vi "Warn.vi"(8 "NwarnIN":bool, 9 "HwarnIN":bool, 10 "warncontN":T1={"alarmliqN"=90.0, "warn?N"=FALSE, "lessthan?N"=FALSE}, 11 "warncontHe":T2={"alarmliqHe"=85.0, "warn?He"=FALSE, "lessthan?He"=FALSE}) -> (2 "warnNOUT":T1={"alarmliqN"=90.0, "warn?N"=FALSE, "lessthan?N"=FALSE}, 3 "warnHeOUT":T2={"alarmliqHe"=85.0, "warn?He"=FALSE, "lessthan?He"=FALSE})   [LabVIEW 2009, in "Level Meter.lvclass"]
uses:
  Level Meter.lvclass
  Global/Sound Files.vi
panel:
  in  "turnoff":bool
  out "Nwarn":bool caption="LN"
  out "Hwarn":bool caption="LHe"
  in  "exit":bool
  out "disp":string
  out "warn2":bool
  out "warn1":bool
  # "Off"
  # "On"
  # "Greater"
  # "Less"
  # "Off"
  # "On"
  # "Greater"
  # "Less"
  # "Off"
  # "On"
  # "Greater"
  # "Less"
  # "Off"
  # "On"
  # "Greater"
  # "Less"
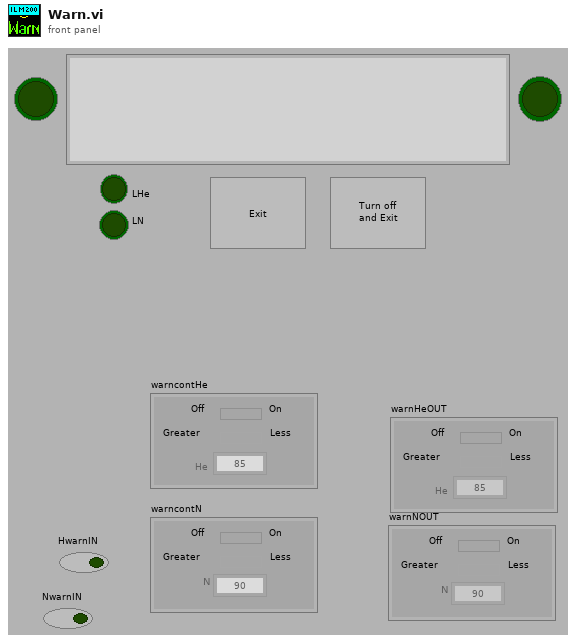
[diagram p1: front panel]
types:
  T1 = cluster{"alarmliqN":dbl, "warn?N":bool, "lessthan?N":bool}
  T2 = cluster{"alarmliqHe":dbl, "warn?He":bool, "lessthan?He":bool}
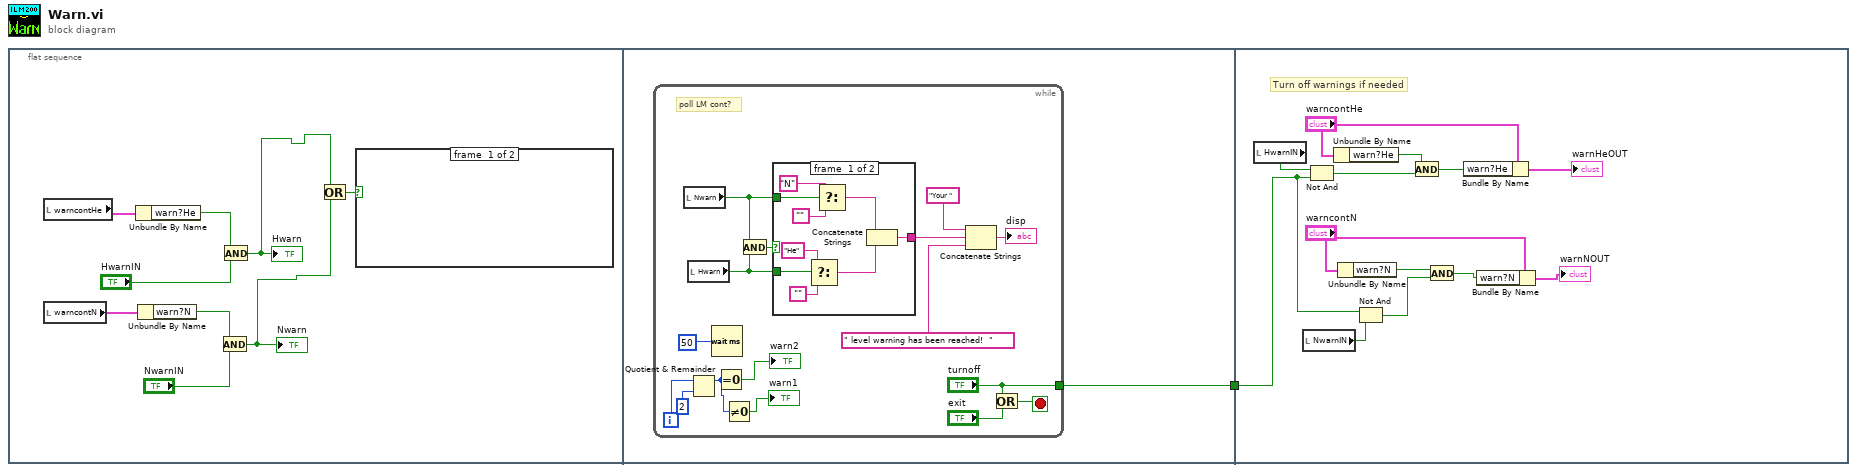
[diagram p0: block diagram]
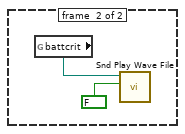
[diagram p2: hidden frame]
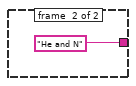
[diagram p3: hidden frame]
diagram:
  n1 = flat-sequence {
    tunnel: [w13] -> w1
    tunnel: w1 -> [w42]
    frame #0 {
      n2 = local read "warncontHe"() -> (w10:T2)
      n3 = local read "warncontN"() -> (w6:T1)
      n4 = Unbundle By Name(w10) -> ("warn?He"=w9:bool)
      n5 = Unbundle By Name(w6) -> ("warn?N"=w7:bool)
      n6 = And(x=w7, y="NwarnIN") -> (x .and. y?=w2:bool)
      "Nwarn" <- w2
      n7 = And(x=w9, y="HwarnIN") -> (x .and. y?=w3:bool)
      "Hwarn" <- w3
      n8 = Or(x=w3, y=w2) -> (x .or. y?=w4:bool)
      n9 = case shown="True" w4 {
        frame #0 {
        }
        frame #1 {
          n10 = global read "Sound Files.vi" "battcrit"() -> (w11:path)
          n11 = call <vilib>:"Snd Play Wave File.vi"("wait until finish (T)"=FALSE, "wave file path"=w11) -> ()  [unwired: 1 in, 9 out]
        }
      }
    }
    frame #1 {
      n12 = while {
        tunnel: ["turnoff"] -> w13
        i -> [w29]
        stop <- w18 stop-if-true
        # "poll LM cont?"
        n13 = local read "Nwarn"() -> (w25:bool)
        n14 = local read "Hwarn"() -> (w24:bool)
        n15 = Quotient & Remainder(x=w29, y=2) -> (x-y*floor(x/y)=w16:i32)  [unwired: 1 out]
        n16 = Wait (ms)(milliseconds to wait=50) -> ()  [unwired: 1 out]
        n17 = Equal To 0?(x=w16) -> (x = 0?=→"warn2":bool)
        n18 = Not Equal To 0?(x=w16) -> (x != 0?=→"warn1":bool)
        n19 = And(x=w25, y=w24) -> (x .and. y?=w26:bool)
        n20 = case shown="False" w26 {
          tunnel: w25 -> [w38 _]
          tunnel: w24 -> [w37 _]
          tunnel: [w30 "He and N"] -> w23
          frame #0 {
            n21 = Select(t="He", s=w37, f="") -> (s? t:f=w36:string)
            n22 = Select(t="N", s=w38, f="") -> (s? t:f=w35:string)
            n23 = Concatenate Strings(w35, w36) -> (w30:string)
          }
          frame #1 {
          }
        }
        n24 = Concatenate Strings("Your ", w23, " level warning has been reached!  ") -> (→"disp":string)
        n25 = Or(x="turnoff", y="exit") -> (x .or. y?=w18:bool)
      }
    }
    frame #2 {
      # "Turn off warnings if needed"
      n26 = local read "HwarnIN"() -> (w40:bool)
      n27 = local read "NwarnIN"() -> (w43:bool)
      n28 = Not And(1:w42, 2:w40) -> (0:w46:bool)
      n29 = Unbundle By Name("warncontHe") -> ("warn?He"=w48:bool)
      n30 = Unbundle By Name("warncontN") -> ("warn?N"=w45:bool)
      n31 = Not And(1:w43, 2:w42) -> (0:w41:bool)
      n32 = And(x=w48, y=w46) -> (x .and. y?=w47:bool)
      n33 = And(x=w45, y=w41) -> (x .and. y?=w44:bool)
      n34 = Bundle By Name(cluster="warncontHe", "warn?He"=w47) -> (→"warnHeOUT":T2)
      n35 = Bundle By Name(cluster="warncontN", "warn?N"=w44) -> (→"warnNOUT":T1)
    }
  }
